vi "Create Start Test Command.vi"(7 "Tx/Rx":T2, 8 "error in (no error)":errorcluster, 9 "Tx Packet Type":T1, 10 "BLE  Channel (Decimal)":u16 max=39) -> (0 "error out":errorcluster, 2 "VISA Hex Cmd":string)   [LabVIEW 2026, in "Nordic nRF52 DK DTM Test.lvlib"]
uses:
  Nordic nRF52 DK DTM Test.lvlib
  TxRx.ctl
  PacketType.ctl
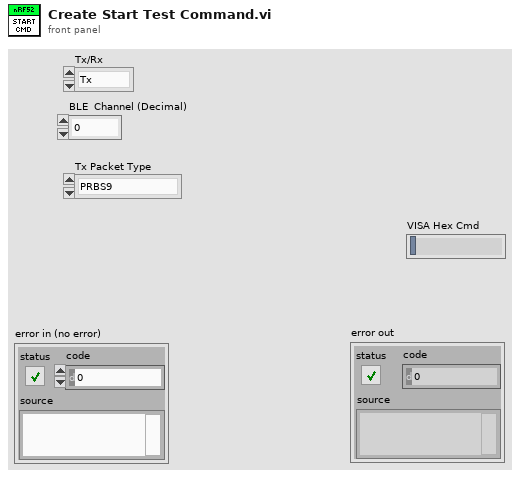
[diagram p1: front panel]
types:
  T1 = typedef "Nordic nRF52 DK DTM Test.lvlib/PacketType.ctl" = enum16{"PRBS9", "DF1", "DF2"}
  T2 = typedef "Nordic nRF52 DK DTM Test.lvlib/TxRx.ctl" = enum16{"Tx", "Rx"}
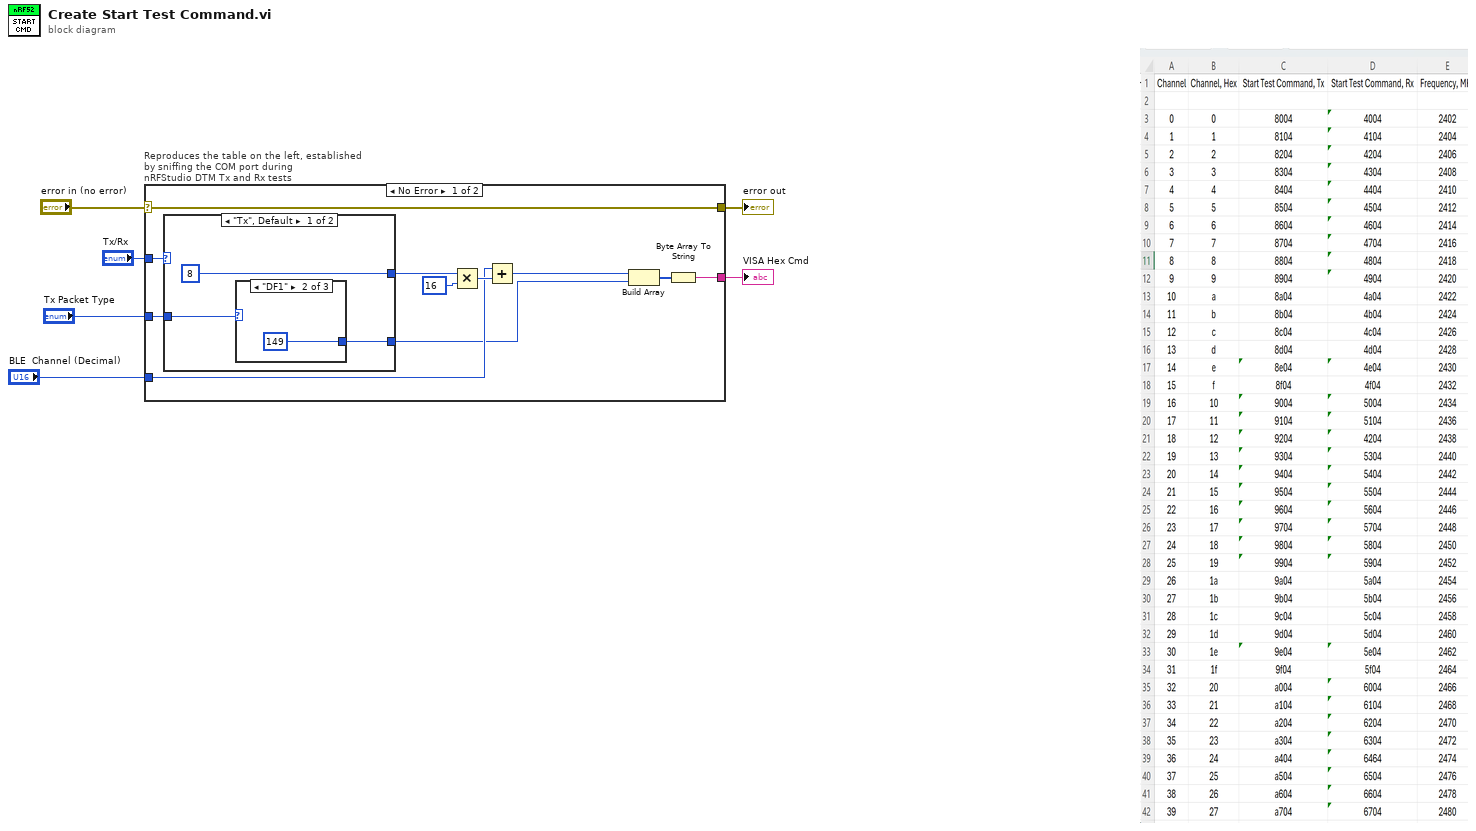
[diagram p0: block diagram]
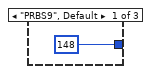
[diagram p2: hidden frame]
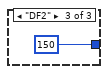
[diagram p3: hidden frame]
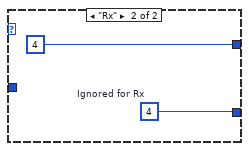
[diagram p4: hidden frame]
diagram:
  n1 = case "Reproduces the table on the left, established by sniffing the COM port during\nnRFStudio DTM Tx and Rx tests" shown="No Error" "error in (no error)" {
    selector: "error in (no error)" -> [w13 w26]
    tunnel: "Tx/Rx" -> [w17 _]
    tunnel: "BLE  Channel (Decimal)" -> [w12 _]
    tunnel: [w13 w26] -> w3
    tunnel: [w10 _] -> w2
    tunnel: "Tx Packet Type" -> [w8 _]
    frame No Error {
      n2 = case shown="\"Tx\", Default" w17 {
        tunnel: [u16 8 u16 4] -> w16
        tunnel: w8 -> [w19 _]
        tunnel: [w18 w24] -> w7
        frame "Tx", Default {
          n3 = case shown="\"DF1\"" w19 {
            tunnel: [u16 148 ("y") u16 149 ("y") u16 150 ("y")] -> w18
            frame "PRBS9", Default {
            }
            frame "DF1" {
            }
            frame "DF2" {
            }
          }
        }
        frame "Rx" {
          w24 = u16 4  # Ignored for Rx
        }
      }
      n4 = Multiply(x=w16, y=u16 16) -> (x*y=w14:u16)
      n5 = Add(x=w12, y=w14) -> (x+y=w9:u16)
      n6 = Build Array(w9, w7) -> (w11:u16[])
      n7 = Byte Array To String(unsigned byte array=w11) -> (string=w10:string)
    }
    frame Error {
    }
  }
  "error out" <- w3
  "VISA Hex Cmd" <- w2
